vi "Shutdown.vi"(7 "Abort":bool, 8 "error in (no error)":errorcluster, 11 "Mediator in":refnum<class "Mediator.lvclass">) -> (0 "error out":errorcluster)   [LabVIEW 2015, in "Mediator.lvlib" / "Mediator.lvclass"]
doc: "This shuts down the Mediator and all associated resources."
uses:
  Mediator.lvclass
  Mediator.lvclass/Mediator.ctl
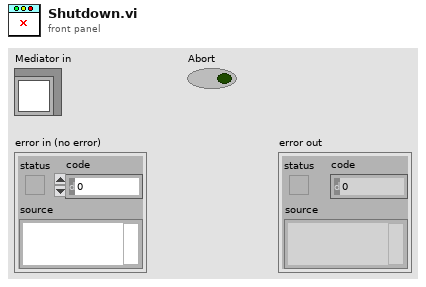
[diagram p1: front panel]
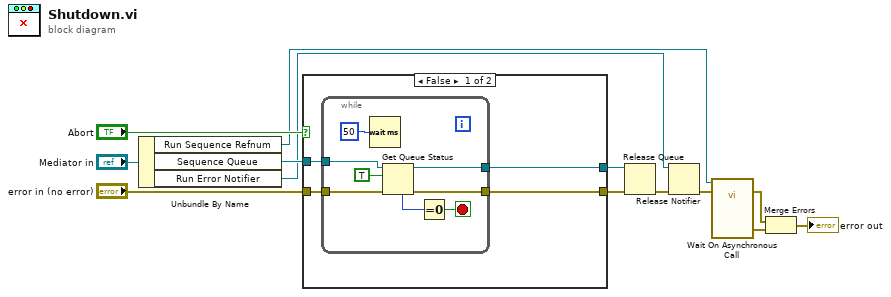
[diagram p0: block diagram]
diagram:
  n1 = Unbundle By Name("Mediator in") -> ("Run Sequence Refnum"=w7:refnum<vi>, "Sequence Queue"=w12:refnum<queue>, "Run Error Notifier"=w3:refnum<notifier>)
  n2 = case shown="False" "Abort" {
    tunnel: w12 -> [w17 w26]
    tunnel: [w16 w26] -> w10
    tunnel: [w14 w27] -> w8
    tunnel: "error in (no error)" -> [w15 w27]
    frame False {
      n3 = while {
        tunnel: w17 -> [w25]
        tunnel: [w22] -> w16
        tunnel: [w21] -> w14
        tunnel: w15 -> [w20]
        stop <- w24 stop-if-true
        n4 = Wait (ms)(milliseconds to wait=u32 50) -> ()  [unwired: 1 out]
        n5 = Get Queue Status(queue=w25, return elements? (F)=TRUE, error in (no error)=w20) -> (queue out=w22:refnum<queue>, error out=w21:errorcluster, # elements in queue=w18:i32)  [unwired: 5 out]
        n6 = Equal To 0?(x=w18) -> (x = 0?=w24:bool)
      }
    }
    frame True {
    }
  }
  n7 = Release Queue(queue=w10, error in (no error)=w8) -> (error out=w2:errorcluster)  [unwired: 1 in, 2 out]
  n8 = Release Notifier(notifier=w3, error in (no error)=w2) -> (error out=w1:errorcluster)  [unwired: 1 in, 2 out]
  n9 = call-by-ref "Wait On Asynchronous Call"(reference=w7, error in=w1) -> (error out=w6:errorcluster, 0:"error out"=w5:errorcluster)  [unwired: 11 in, 1 out]
  n10 = Merge Errors(w6, w5) -> (→"error out":errorcluster)
